vi "host.vi"() -> ()   [LabVIEW 2020]
uses:
  <vilib>/FPGAPlugInAG/cRIO-9035/niLvFpga_Open_cRIO-9035.vi
  <vilib>/rvi/interface/common/dynamic/niFpgaDynamicAddResources.vi
  <vilib>/Utility/error.llb/Error Cluster From Error Code.vi
  <vilib>/rvi/errors/niLvFpgaAdjustHostInterfaceError.vi
  <vilib>/FPGAPlugInAG/Dynamic/niLvFpga_Run_Dynamic.vi
  <vilib>/FPGAPlugInAG/Dynamic/niLvFpga_Close_Dynamic.vi
  <vilib>/rvi/interface/nirviOpenFPGA/nirviOpenFPGA.xnode
  FPGA Bitfiles/v1.1_FPGATarget_target_EWXeUKZodsc.lvbitx
  target.vi
  <vilib>/rvi/interface/nirviMethod/nirviMethod.xnode
  <vilib>/rvi/interface/nirviReadWriteControl/nirviReadWriteControl.xnode
  <vilib>/rvi/interface/nirviCloseFPGA/nirviCloseFPGA.xnode
  <vilib>/rvi/errors/niLvFpgaMergeErrorWithErrorCode.vi
  <vilib>/FPGAPlugInAG/Dynamic/niLvFpga_WriteFifo_Dynamic.vi
  <vilib>/FPGAPlugInAG/Dynamic/niLvFpga_ReadFifo_Dynamic.vi
  NiFpgaLv.dll
  <vilib>/rvi/interface/Simulation/niFpgaSimulationCallBeginRW.vi
panel:
  out "n out":i32
  out "m out":i32
  out "sum of error":dbl
  out "B - FPGA code":sgl[][](array[numeric])
  out "B - Real":dbl[][](array[numeric])
  out "A":sgl[][](array[numeric])
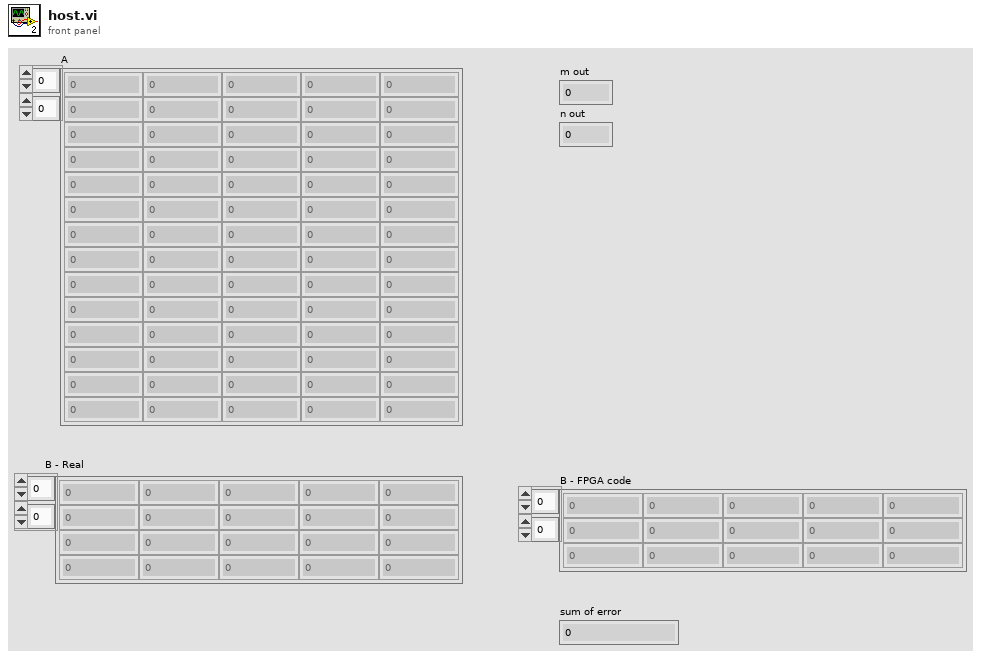
[diagram p1: front panel]
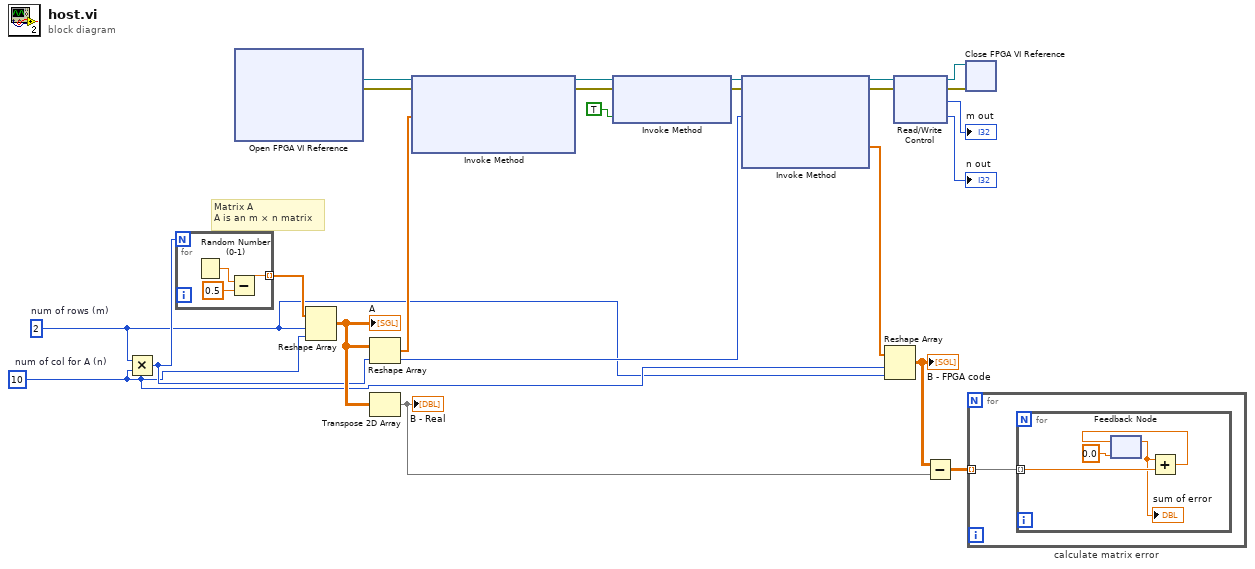
[diagram p0: block diagram]
diagram:
  w8 = 10  # num of col for A (n)
  w7 = 2  # num of rows (m)
  # "Matrix A\nA is an m × n matrix"
  n1 = Multiply(x=w7, y=w8) -> (x*y=w12:i32)
  n2 = for {
    N: w12 -> [_]
    tunnel: [w25] -> w18 mode=indexing
    n3 = Random Number (0-1)() -> (number: 0 to 1=w26:dbl)
    n4 = Subtract(x=w26, y=sgl 0.5) -> (x-y=w25:sgl)
  }
  n5 = xnode "Open FPGA VI Reference"() -> ("FPGA VI Reference Out"=w22:refnum<k20>, "error out"=w21:errorcluster)  [unwired: 2 in]
  n6 = Reshape Array(w18, w7, w8) -> (w14:sgl[][])
  "A" <- w14
  n7 = Reshape Array(w14, w12) -> (w17:sgl[])
  n8 = Transpose 2D Array(2D array=w14) -> (transposed array=w13:sgl[][])
  "B - Real" <- w13
  n9 = xnode "Invoke Method"("FPGA VI Reference In"=w22, "error in"=w21, "Data"=w17) -> ("FPGA VI Reference Out"=w11:refnum<k20>, "error out"=w10:errorcluster)  [unwired: 1 in, 1 out]
  n10 = xnode "Invoke Method"("FPGA VI Reference In"=w11, "error in"=w10, "Wait Until Done (F)"=TRUE) -> ("FPGA VI Reference Out"=w20:refnum<k20>, "error out"=w19:errorcluster)
  n11 = xnode "Invoke Method"("FPGA VI Reference In"=w20, "error in"=w19, "Number of Elements"=w12) -> ("FPGA VI Reference Out"=w6:refnum<k20>, "error out"=w2:errorcluster, "Data"=w15:sgl[])  [unwired: 1 in, 1 out]
  n12 = Reshape Array(w15, w8, w7) -> (w9:sgl[][])
  "B - FPGA code" <- w9
  n13 = xnode "Read/Write Control"("FPGA VI Reference In"=w6, "error in"=w2) -> ("FPGA VI Reference Out"=w3:refnum<k20>, "error out"=w1:errorcluster, "m"=→"m out":i32, "n"=→"n out":i32)
  n14 = Subtract(x=w9, y=w13) -> (x-y=w16:sgl[][])
  n15 = xnode "Close FPGA VI Reference"("FPGA VI Reference In"=w3, "error in"=w1) -> ()  [unwired: 1 out]
  n16 = for "calculate matrix error" {
    tunnel: w16 -> [w27] mode=indexing
    n17 = for {
      tunnel: w27 -> [w31] mode=indexing
      n18 = feedback #1(0.0) -> (w29:dbl)
      "sum of error" <- w29
      n19 = Add(x=w29, y=w31) -> (x+y=w30:dbl)
      n20 = feedback-in #1(w30) -> ()
    }
  }
